vi "UE9 PWM and Quadrature.vi"(8 "error in":errorcluster, 9 "PWM16 Duty Cycle [%]":dbl=50.0 format="%.1f") -> (2 "Quadrature Count":i32)   [LabVIEW 2021]
panel:
  out "aUpdateResetTimers":bool[](array[boolean])
  in  "Reset Quadrature Count":bool
  out "Timer Value Array":u16[](array[numeric])
  in  "stop":bool
  in  "FirstFound":bool=TRUE
  in  "Address":string="1"
  in  "ConnectionType":u16(ring) items=["LJ_ctUSB", "LJ_ctETHERNET"]
  out "Error Message":string
  # "Demonstrates 1 quadrature pair (FIO0 & FIO1) with 1 PWM16 output (FIO2)."
  # "This VI allows the duty cycle to\nbe changed while the VI is running."
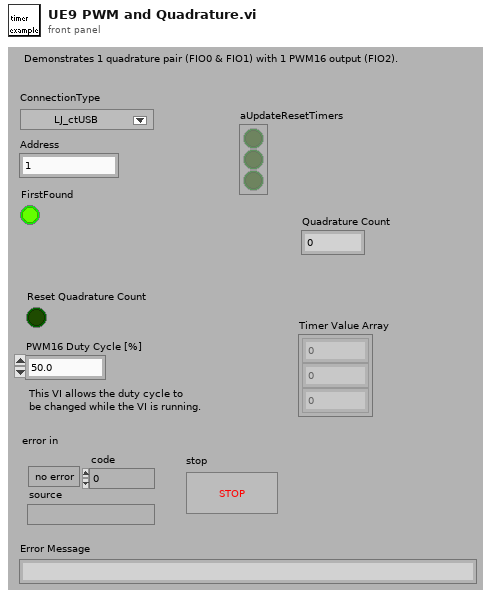
[diagram p1: front panel]
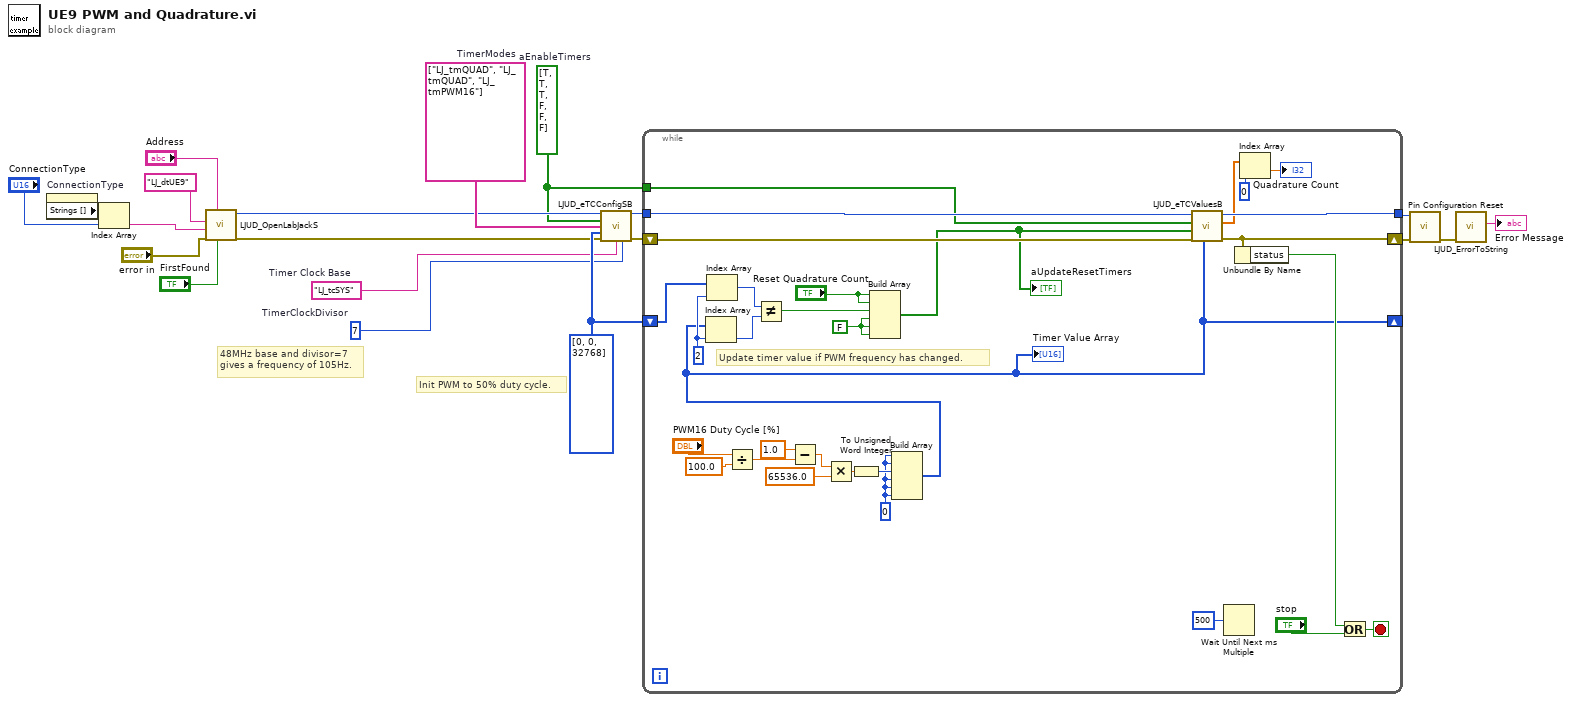
[diagram p0: block diagram]
diagram:
  w1 = 7  # TimerClockDivisor
  w3 = "LJ_tcSYS"  # Timer Clock Base
  w2 = bool[] [TRUE, TRUE, TRUE, FALSE, FALSE, FALSE]  # aEnableTimers
  w6 = string[] ["LJ_tmQUAD", "LJ_tmQUAD", "LJ_tmPWM16"]  # TimerModes
  w10 = u16[] [0, 0, 32768] ("TimerValues")
  # "48MHz base and divisor=7\ngives a frequency of 105Hz."
  # "Init PWM to 50% duty cycle."
  n1 = property on="ConnectionType" class="Ring (strict)"() -> ("Strings []"=w15:string[])  [unwired: 2 in, 2 out]
  n2 = Index Array(array=w15, index="ConnectionType") -> (element=w13:string)
  n3 = call "LJUD_OpenLabJackS.vi"("FirstFound"="FirstFound", "Address"="Address", "error in"="error in", "ConnectionType"=w13, "DeviceType"="LJ_dtUE9") -> ("error out"=w4:errorcluster, "Handle"=w5:i32)  [unwired: 4 in, 1 out]
  n4 = call "LJUD_eTCConfigSB.vi"("Handle In"=w5, "aEnableTimers"=w2, "aTimerModes"=w6, "aTimerValues"=w10, "error in"=w4, "TimerClockBase"=w3, "TimerClockDivisor"=w1) -> ("Handle Out"=w12:i32, "error out"=w11:errorcluster)  [unwired: 7 in]
  n5 = while {
    tunnel: w2 -> [w42]
    tunnel: [w46] -> w9
    shift-left: w10 -> [w35]
    shift-right: [w22] -> _
    tunnel: w12 -> [w49]
    shift-left: w11 -> [w50]
    shift-right: [w47] -> w8
    stop <- w48 stop-if-true
    w24 = FALSE ("Input Element")
    w26 = u16 0 ("PWM Timer Value")
    w41 = 2 ("Index")
    # "Update timer value if PWM frequency has changed."
    n6 = Index Array(array=w35, index=w41) -> (element=w40:u16)
    n7 = Divide(x="PWM16 Duty Cycle [%]", y=100.0) -> (x/y=w32:dbl)
    n8 = Subtract(x=1.0, y=w32) -> (x-y=w30:dbl)
    n9 = Multiply(x=w30, y=65536.0) -> (x*y=w29:dbl)
    n10 = To Unsigned Word Integer(number=w29) -> (unsigned 16bit integer=w27:u16)
    n11 = Build Array(w26, w26, w27, w26, w26, w26) -> (w22:u16[])
    "Timer Value Array" <- w22
    n12 = Index Array(array=w22, index=w41) -> (element=w39:u16)
    n13 = Not Equal?(x=w40, y=w39) -> (x != y?=w21:bool)
    n14 = Build Array("Reset Quadrature Count", "Reset Quadrature Count", w21, w24, w24, w24) -> (w23:bool[])
    "aUpdateResetTimers" <- w23
    n15 = call "LJUD_eTCValuesB.vi"("aTimerValues Write"=w22, "error in"=w50, "aUpdateResetTimers"=w23, "aReadTimers"=w42, "Handle In"=w49) -> ("error out"=w47:errorcluster, "aTimerValues Read"=w37:dbl[], "Handle Out"=w46:i32)  [unwired: 3 in, 1 out]
    n16 = Wait Until Next ms Multiple(millisecond multiple=u32 500) -> ()  [unwired: 1 out]
    n17 = Unbundle By Name(w47) -> ("status"=w45:bool)
    n18 = Index Array(array=w37, index=0 ("Index")) -> (element=→"Quadrature Count":dbl)
    n19 = Or(x=w45, y="stop") -> (x .or. y?=w48:bool)
  }
  n20 = call "Pin Configuration Reset.vi"("error in"=w8, "Handle In"=w9) -> ("error out"=w7:errorcluster)  [unwired: 8 in, 1 out]
  n21 = call "LJUD_ErrorToString.vi"("error in"=w7) -> ("String"=→"Error Message":string)  [unwired: 10 in]
